vi "Construct.vi"(6 "channels":u8[](array[numeric]), 8 "error in":errorcluster, 11 "identifier":string) -> (0 "error out":errorcluster, 3 "logging execution unit out":refnum<class "Logging Execution Unit.lvclass">)   [LabVIEW 2020, in "AIM ARINC 429 Engine.lvlib" / "Implementation.lvlib" / "Logging Execution Unit.lvclass"]
uses:
  Logging Execution Unit.lvclass
  Custom Device/Hardware Handles.ctl
  Custom Device/Custom Device.lvlib
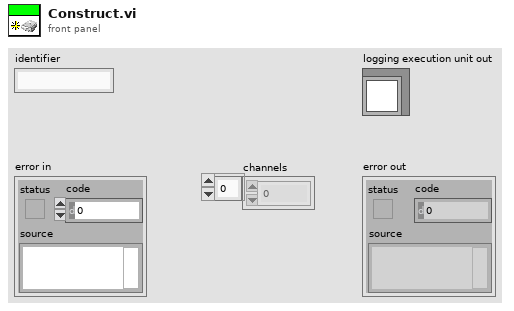
[diagram p1: front panel]
types:
  T1 = typedef "AIM ARINC 429 Engine.lvlib/Custom Device.lvlib/Hardware Handles.ctl" = cluster{"module":u8}
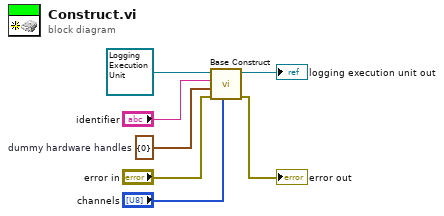
[diagram p0: block diagram]
diagram:
  w4 = T1 {"module"=0}  # dummy hardware handles
  n1 = call-dynamic "Base Construct.vi"("channels"="channels", "error in"="error in", "hardware handles"=w4, "identifier"="identifier", "execution unit in"=refnum<class "Logging Execution Unit.lvclass"> refnum ("Logging Execution Unit out")) -> ("error out"=→"error out":errorcluster, "execution unit out"=→"logging execution unit out":refnum<class "Logging Execution Unit.lvclass">)  [unwired: 5 in]
